vi "ACK Subscriptions Publications.vi"(0 "GEA2 Reference In":refnum<k24>, 7 "GEA2 Msg":T1 {"Command" format="%02x"; "Destination" format="%02x"; "Source" format="%02x"}, 11 "error in (no error)":errorcluster) -> (4 "GEA2 Reference Out":refnum<k24>, 15 "error out":errorcluster)   [LabVIEW 2021]
uses:
  Common/LabVIEW GEA2 Toolkit/GEA3/type defs/Data In.ctl
  D:/Common/LabVIEW GEA2 Toolkit/source/GEA3 DLL Source/GeaCommunication.dll
  Common/LabVIEW GEA2 Toolkit/source/GEA3 DLL Source/GeaCommunication.dll
  Common/LabVIEW GEA2 Toolkit/GEA3/library/GEA2_Toolkit.lvlib
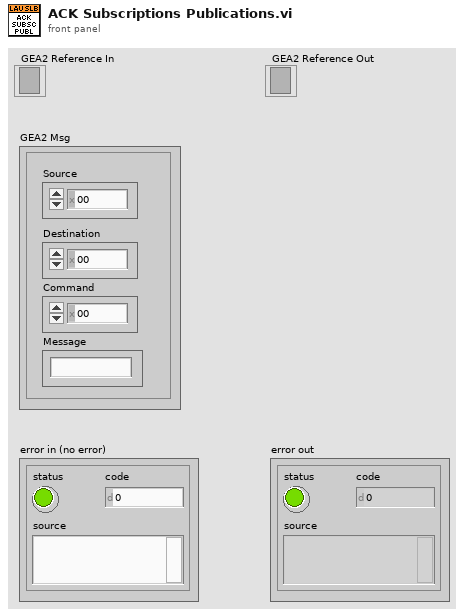
[diagram p1: front panel]
types:
  T1 = typedef "Data In.ctl" = cluster{"Source":u8, "Destination":u8, "Command":u8, "Message":string}
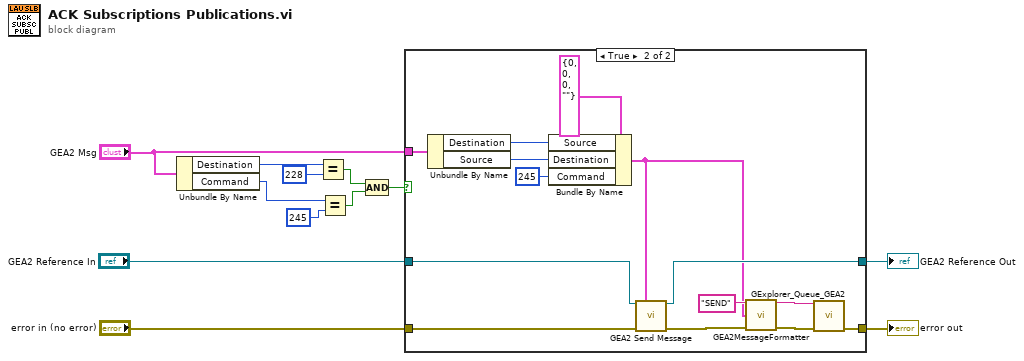
[diagram p0: block diagram]
diagram:
  n1 = Unbundle By Name("GEA2 Msg") -> ("Destination"=w8:u8, "Command"=w5:u8)
  n2 = Equal?(x=w8, y=u8 228) -> (x = y?=w7:bool)
  n3 = Equal?(x=w5, y=u8 245) -> (x = y?=w3:bool)
  n4 = Compound Arithmetic op=AND(w7, w3) -> (w12:bool)
  n5 = case shown="True" w12 {
    tunnel: "error in (no error)" -> [w14 w28]
    tunnel: [w14 w16] -> w11
    tunnel: "GEA2 Msg" -> [_ w27]
    tunnel: "GEA2 Reference In" -> [w13 w22]
    tunnel: [w13 w21] -> w1
    frame False {
    }
    frame True {
      n6 = Unbundle By Name(w27) -> ("Destination"=w23:u8, "Source"=w25:u8)
      n7 = Bundle By Name(cluster=T1 {"Source"=0, "Destination"=0, "Command"=0, "Message"=""} ("GEA2 Msg"), "Source"=w23, "Destination"=w25, "Command"=u8 245) -> (w15:T1)
      n8 = call "GEA2 Send Message.vi"("GEA2 Reference In"=w22, "Input Data"=w15, "Error In"=w28) -> ("GEA2 Reference Out"=w21:refnum<k24>, "Error Out"=w17:errorcluster)  [unwired: 11 in]
      n9 = call "GEA2MessageFormatter.vi"("Prefix(Send/Recv)"="SEND", "GEA2 Data In"=w15, "Error In"=w17) -> ("Output String"=w18:string, "Error Out"=w19:errorcluster)  [unwired: 11 in]
      n10 = call "GExplorer_Queue_GEA2.vi"("Output String"=w18, "error in (no error)"=w19) -> ("error out"=w16:errorcluster)  [unwired: 13 in]
    }
  }
  "error out" <- w11
  "GEA2 Reference Out" <- w1
